vi "개별쓰기요구(subVI).vi"(1 "데이터":u16[](array[numeric])=[13106, 13104, 13107, 13108, 9521, 12848, 13620, 13879] format="%.0x", 2 "변수이름 배열":string[](array[string])) -> (0 "개별쓰기":string)   [LabVIEW 2014]
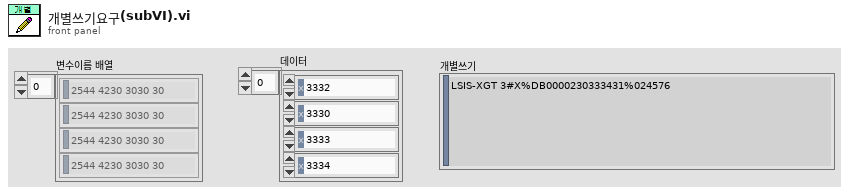
[diagram p1: front panel]
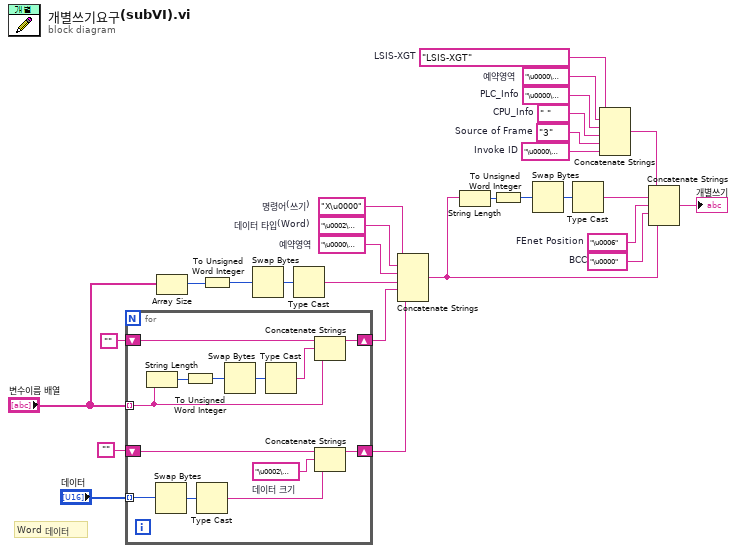
[diagram p0: block diagram]
diagram:
  w17 = "\u0000"  # BCC
  w18 = "\u0006"  # FEnet Position
  w20 = "\u0000\u0000"  # Invoke ID
  w21 = "3"  # Source of Frame
  w22 = " "  # CPU_Info
  w23 = "\u0000\u0000"  # PLC_Info
  w24 = "\u0000\u0000"  # 예약영역
  w25 = "LSIS-XGT"  # LSIS-XGT
  w11 = "\u0000\u0000"  # 예약영역
  w27 = "\u0002\u0000"  # 데이터 타입(Word)
  w28 = "X\u0000"  # 명령어(쓰기)
  # "Word 데이터"
  n1 = for {
    tunnel: "변수이름 배열" -> [w35] mode=indexing
    shift-right: [w37] -> w4
    shift-left: "" -> [w38]
    shift-right: [w31] -> w1
    shift-left: "" -> [w32]
    tunnel: "데이터" -> [w33] mode=indexing
    w30 = "\u0002\u0000"  # 데이터 크기
    n2 = String Length(string=w35) -> (length=w39:i32)
    n3 = Swap Bytes(anything=w33) -> (byte swapped=w34:u16)
    n4 = To Unsigned Word Integer(number=w39) -> (unsigned 16bit integer=w40:u16)
    n5 = Type Cast(x=w34) -> (*(type *) &x=w29:string)  [unwired: 1 in]
    n6 = Swap Bytes(anything=w40) -> (byte swapped=w41:u16)
    n7 = Type Cast(x=w41) -> (*(type *) &x=w36:string)  [unwired: 1 in]
    n8 = Concatenate Strings(w38, w36, w35) -> (w37:string)
    n9 = Concatenate Strings(w32, w30, w29) -> (w31:string)
  }
  n10 = Array Size(array="변수이름 배열") -> (size(s)=w8:i32)
  n11 = To Unsigned Word Integer(number=w8) -> (unsigned 16bit integer=w9:u16)
  n12 = Swap Bytes(anything=w9) -> (byte swapped=w10:u16)
  n13 = Type Cast(x=w10) -> (*(type *) &x=w7:string)  [unwired: 1 in]
  n14 = Concatenate Strings(w28, w27, w11, w7, w4, w1) -> (w19:string)
  n15 = String Length(string=w19) -> (length=w26:i32)
  n16 = To Unsigned Word Integer(number=w26) -> (unsigned 16bit integer=w15:u16)
  n17 = Swap Bytes(anything=w15) -> (byte swapped=w14:u16)
  n18 = Type Cast(x=w14) -> (*(type *) &x=w13:string)  [unwired: 1 in]
  n19 = Concatenate Strings(w25, w24, w23, w22, w21, w20) -> (w12:string)
  n20 = Concatenate Strings(w12, w13, w18, w17, w19) -> (→"개별쓰기":string)
